vi "BoxGetNoteState.vi"() -> (0 "Box Note State":T1)   [LabVIEW 2023]
uses:
  BoxNoteState.ctl
  BoxGlobals.vi
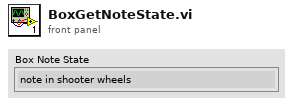
[diagram p1: front panel]
types:
  T1 = typedef "BoxNoteState.ctl" = enum16{"note in shooter wheels", "misaligned note", "no note", "have note"}
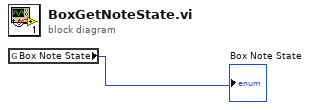
[diagram p0: block diagram]
diagram:
  n1 = global read "BoxGlobals.vi" "Box Note State"() -> (→"Box Note State":T1)
